vi "Get Full Config.vi"(8 "error in (no error)":errorcluster, 11 "Device in":refnum<class "Device.lvclass">) -> (0 "error out":errorcluster, 1 "Config Values":string[](array[string]), 2 "Config Keys":string[](array[string]), 3 "Device out":refnum<class "Device.lvclass">)   [LabVIEW 2020, in "HAL.lvlib" / "Device.lvclass"]
uses:
  Device.lvclass
  Device.lvclass/Device.ctl
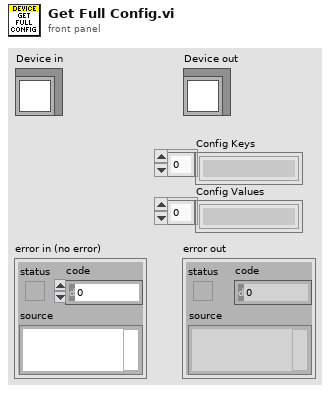
[diagram p1: front panel]
types:
  T1 = typedef "HAL.lvlib/Device.lvclass/Ref Data.ctl" = cluster{"Config Keys":string[], "Config Values":string[], "Cal Expires":timestamp, "Name":string, "Comment":string, "State":T2, "Error":errorcluster}
  T2 = typedef "HAL.lvlib/Device.lvclass/Device State.ctl" = enum16{"Uninitialized", "Initialized", "Running", "Error"}
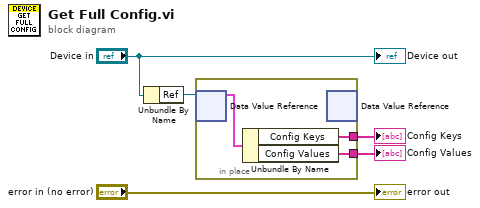
[diagram p0: block diagram]
diagram:
  n1 = Unbundle By Name("Device in") -> ("Ref"=w4:refnum<data-value>)
  n2 = in-place {
    in-place-border: [w7] -> w2
    in-place-border: [w6] -> w1
    n3 = in-place-dvr #1(w4) -> (w8:T1)  [unwired: 1 out]
    n4 = Unbundle By Name(w8) -> ("Config Keys"=w7:string[], "Config Values"=w6:string[])
    n5 = in-place-dvr #1() -> ()  [unwired: 1 in, 2 out]
  }
  "Config Keys" <- w2
  "Config Values" <- w1
  "error out" <- "error in (no error)"
  "Device out" <- "Device in"
